vi "_convertInput.vi"(0 "pry":dbl[](array[numeric]), 3 "FBLR":dbl[](array[numeric])) -> (7 "FBLR":dbl[](array[numeric]), 10 "pry":dbl[](array[numeric]))   [LabVIEW 2021, in "System.lvclass"]
uses:
  System.lvclass
  <vilib>/Analysis/baseanly.llb/A x B.vi
  <vilib>/Analysis/baseanly.llb/Vector x A.vi
  <vilib>/Analysis/Matrix/Numeric/Conversions/Array To Matrix - RA2.vi
  <vilib>/Analysis/NI_AALBase.lvlib
  <vilib>/Analysis/Matrix/NI_Matrix.lvlib
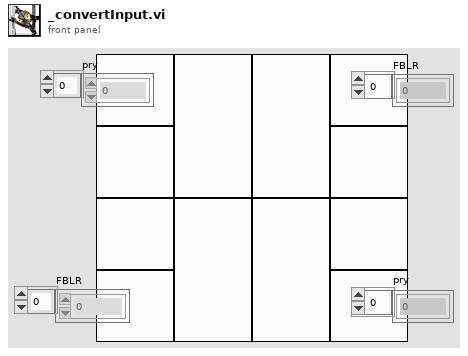
[diagram p1: front panel]
types:
  T1 = typedef "NI_Matrix.lvlib/RealMatrix.ctl" = dbl[][]
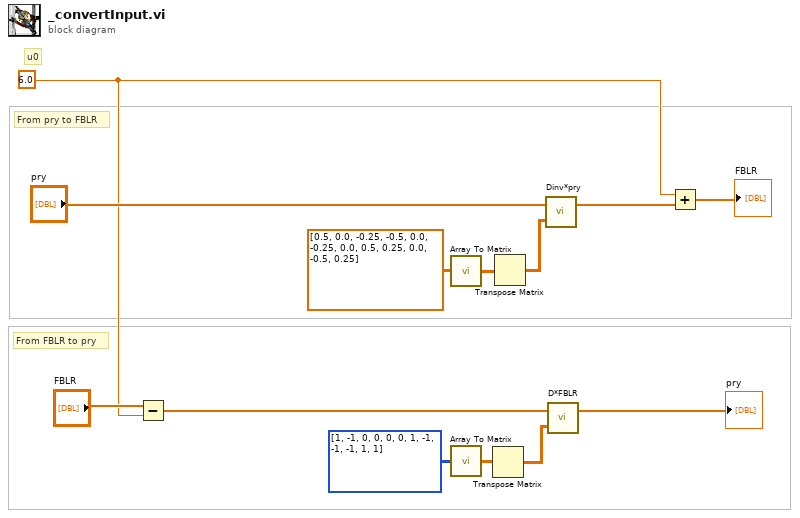
[diagram p0: block diagram]
diagram:
  w7 = 6.0
  # "u0"
  # "From FBLR to pry"
  # "From pry to FBLR"
  n1 = Subtract(x="FBLR", y=w7) -> (x-y=w11:dbl[])
  n2 = call-poly <vilib>:"Array To Matrix.vi"("Real 2D Array"=dbl[][] [[0.5, 0.0, -0.25], [-0.5, 0.0, -0.25], [0.0, 0.5, 0.25], [0.0, -0.5, 0.25]]) -> ("Real Matrix"=w4:T1)
  n3 = call-poly <vilib>:"Array To Matrix.vi"("Real 2D Array"=i32[][] [[1, -1, 0, 0], [0, 0, 1, -1], [-1, -1, 1, 1]]) -> ("Real Matrix"=w2:T1)
  n4 = Transpose Matrix(1:w2) -> (0:w1:T1)
  n5 = Transpose Matrix(1:w4) -> (0:w3:T1)
  n6 = call-poly "Dinv*pry"("Matrix A"=w3, "Vector V'"="pry") -> ("V' x A"=w12:dbl[])  [unwired: 1 out]
  n7 = call-poly "D*FBLR"("Matrix A"=w1, "Vector V'"=w11) -> ("V' x A"=→"pry":dbl[])  [unwired: 1 out]
  n8 = Add ("Add.vi")(x=w7, y=w12) -> (x+y=→"FBLR":dbl[])
